vi "Write Batch Setpoint.vi"(7 "Unit ID (A)":string="A", 8 "error in":errorcluster, 9 "Batch SetPoint":dbl, 10 "Legacy Status":u8(ring)=1 items=["Rev. 21 Board", "Rev. 22 Board", "Rev. 23 Board"], 11 "VISA Session In":refnum<visa-resource-name>="Alicat") -> (0 "error out":errorcluster, 3 "VISA Session Out":refnum<visa-resource-name>)   [LabVIEW 2019]
doc: "Writes a batch setpoint into an Alicat device. ONLY AVAILABLE FOR R22 BOARDS AND ABOVE (run \"Legacy Detector.vi\" to determine board revision), provided that the unit is a controller with totalizer functionality and a firmware version of at least 4v33."
uses:
  <vilib>/Instr/_visa.llb/VISA Flush IO Buffer Mask.ctl
panel:
  # "ONLY AVAILABLE FOR R22 BOARDS AND ABOVE\n(provided it is a controller with totalizer and at least firmware 4v33)"
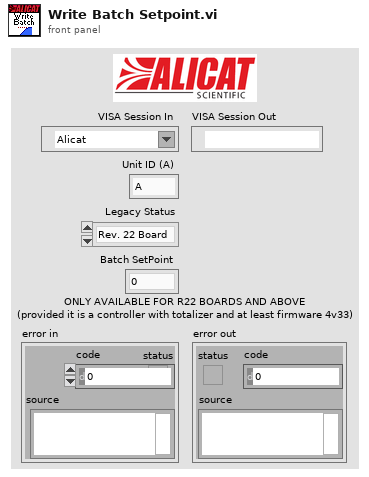
[diagram p1: front panel]
types:
  T1 = typedef "VISA Flush IO Buffer Mask.ctl" = u16
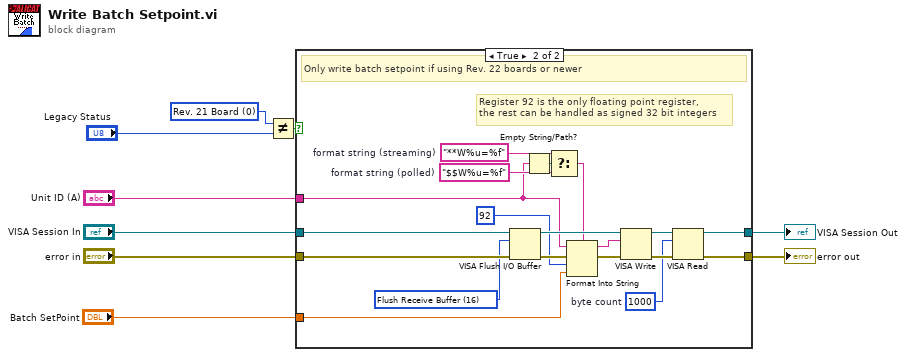
[diagram p0: block diagram]
diagram:
  w3 = u8 0 items=["Rev. 21 Board", "Rev. 22 Board", "Rev. 23 Board"] ("Legacy Status")
  n1 = Not Equal?(x=w3, y="Legacy Status") -> (x != y?=w4:bool)
  n2 = case shown="True" w4 {
    tunnel: "VISA Session In" -> [w11 w29]
    tunnel: "error in" -> [w10 w27]
    tunnel: [w10 w12] -> w7
    tunnel: [w11 w24] -> w6
    tunnel: "Unit ID (A)" -> [_ w15]
    tunnel: "Batch SetPoint" -> [_ w13]
    frame False {
    }
    frame True {
      w16 = "**W%u=%f"  # format string (streaming)
      w18 = "$$W%u=%f"  # format string (polled)
      w26 = T1 16 items=["Flush Receive Buffer"=16, "Write Transmit Buffer to Device"=32, "Flush Receive Buffer (No I/O)"=64, "Flush Transmit Buffer"=128] ("Mask")
      w23 = u32 1000  # byte count
      # "Register 92 is the only floating point register, \nthe rest can be handled as signed 32 bit integers"
      # "Only write batch setpoint if using Rev. 22 boards or newer"
      n3 = VISA Flush I/O Buffer(VISA resource name=w29, mask (16)=w26, error in (no error)=w27) -> (VISA resource name out=w28:refnum<visa-resource-name>, error out=w21:errorcluster)
      n4 = Empty String/Path?(string/path=w15) -> (empty?=w17:bool)
      n5 = Select(t=w16, s=w17, f=w18) -> (s? t:f=w14:string)
      n6 = Format Into String(format string=w14, initial string=w15, error in=w21, u16 92 ("Register address"), w13) -> (resulting string=w22:string, error out=w20:errorcluster)
      n7 = VISA Write(VISA resource name=w28, write buffer=w22, error in (no error)=w20) -> (VISA resource name out=w25:refnum<visa-resource-name>, error out=w30:errorcluster)  [unwired: 1 out]
      n8 = VISA Read(VISA resource name=w25, byte count=w23, error in (no error)=w30) -> (VISA resource name out=w24:refnum<visa-resource-name>, error out=w12:errorcluster)  [unwired: 2 out]
    }
  }
  "error out" <- w7
  "VISA Session Out" <- w6
